vi "Set (SubVI).vi"(8 "Mode":i32, 9 "speed":dbl) -> (0 "Reach?":bool, 1 "Vp":dbl, 2 "Vy":dbl, 3 "Vx":dbl)   [LabVIEW 2017]
uses:
  Projects/Auto control/Inputs.vi
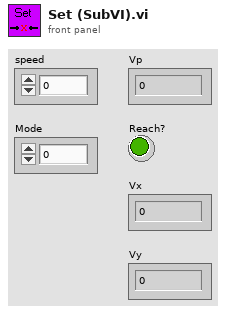
[diagram p1: front panel]
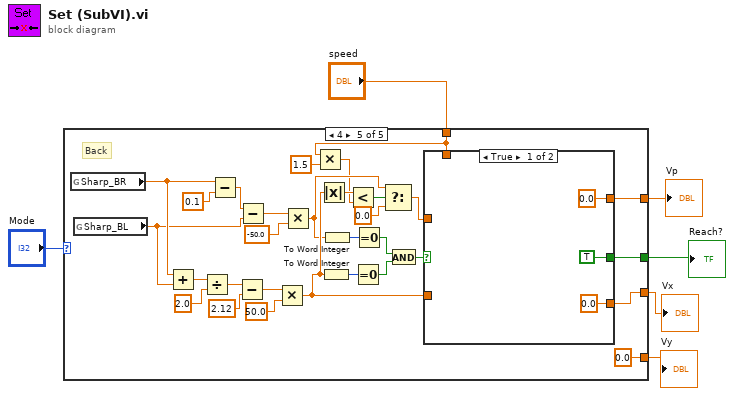
[diagram p0: block diagram]
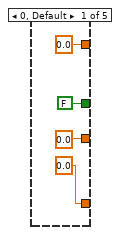
[diagram p2: hidden frame]
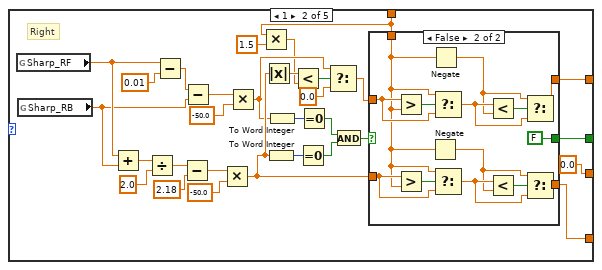
[diagram p3: hidden frame]
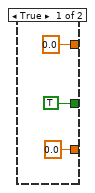
[diagram p4: hidden frame]
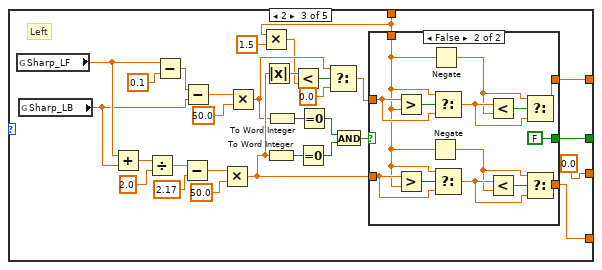
[diagram p5: hidden frame]
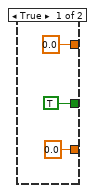
[diagram p6: hidden frame]
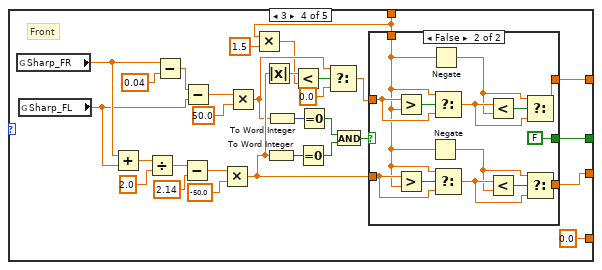
[diagram p7: hidden frame]
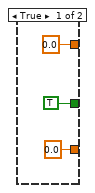
[diagram p8: hidden frame]
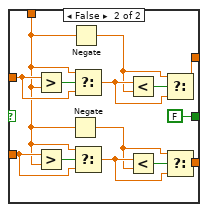
[diagram p9: hidden frame]
diagram:
  n1 = case shown="4" "Mode" {
    tunnel: [0.0 ("speed") w36 w83 w130 w177] -> w2
    tunnel: [0.0 ("speed") 0.0 ("speed") 0.0 ("speed") w106 w153] -> w5
    tunnel: "speed" -> [_ w13 w60 w107 w154]
    tunnel: [FALSE w22 w69 w116 w163] -> w1
    tunnel: [0.0 ("speed") w11 w58 0.0 ("speed") 0.0 ("speed")] -> w6
    frame 0, Default {
    }
    frame 1 {
      # "Right"
      n2 = global read "Inputs.vi" "Sharp_RF"() -> (w35:dbl)
      n3 = global read "Inputs.vi" "Sharp_RB"() -> (w34:dbl)
      n4 = Add(x=w35, y=w34) -> (x+y=w33:dbl)
      n5 = Divide(x=w33, y=2.0) -> (x/y=w31:dbl)
      n6 = Subtract(x=w35, y=0.01) -> (x-y=w40:dbl)
      n7 = Subtract(x=w31, y=2.18) -> (x-y=w29:dbl)
      n8 = Subtract(x=w40, y=w34) -> (x-y=w38:dbl)
      n9 = Multiply(x=w29, y=-50.0) -> (x*y=w18:dbl)
      n10 = Multiply(x=w38, y=-50.0) -> (x*y=w17:dbl)
      n11 = Multiply(x=w13, y=1.5) -> (x*y=w14:dbl)
      n12 = Absolute Value(x=w18) -> (abs(x)=w19:dbl)
      n13 = To Word Integer(number=w18) -> (16bit integer=w26:i16)
      n14 = To Word Integer(number=w17) -> (16bit integer=w27:i16)
      n15 = Less?(x=w19, y=w14) -> (x < y?=w20:bool)
      n16 = Equal To 0?(x=w26) -> (x = 0?=w24:bool)
      n17 = Equal To 0?(x=w27) -> (x = 0?=w23:bool)
      n18 = Select(t=w17, s=w20, f=0.0) -> (s? t:f=w21:dbl)
      n19 = And(x=w23, y=w24) -> (x .and. y?=w25:bool)
      n20 = case shown="False" w25 {
        tunnel: w21 -> [_ w56]
        tunnel: [0.0 ("speed") w52] -> w36
        tunnel: w18 -> [_ w50]
        tunnel: [0.0 ("speed") w46] -> w11
        tunnel: w13 -> [_ w45]
        tunnel: [TRUE FALSE] -> w22
        frame True {
        }
        frame False {
          n21 = Greater?(x=w56, y=w45) -> (0:w57:bool)
          n22 = Greater?(x=w50, y=w45) -> (0:w51:bool)
          n23 = Negate(x=w45) -> (-x=w47:dbl)
          n24 = Negate(x=w45) -> (-x=w53:dbl)
          n25 = Select(t=w45, s=w57, f=w56) -> (s? t:f=w54:dbl)
          n26 = Select(t=w45, s=w51, f=w50) -> (s? t:f=w48:dbl)
          n27 = Less?(x=w54, y=w53) -> (x < y?=w55:bool)
          n28 = Less?(x=w48, y=w47) -> (x < y?=w49:bool)
          n29 = Select(t=w53, s=w55, f=w54) -> (s? t:f=w52:dbl)
          n30 = Select(t=w47, s=w49, f=w48) -> (s? t:f=w46:dbl)
        }
      }
    }
    frame 2 {
      # "Left"
      n31 = global read "Inputs.vi" "Sharp_LF"() -> (w82:dbl)
      n32 = global read "Inputs.vi" "Sharp_LB"() -> (w81:dbl)
      n33 = Add(x=w82, y=w81) -> (x+y=w80:dbl)
      n34 = Divide(x=w80, y=2.0) -> (x/y=w78:dbl)
      n35 = Subtract(x=w82, y=0.1) -> (x-y=w87:dbl)
      n36 = Subtract(x=w78, y=2.17) -> (x-y=w76:dbl)
      n37 = Subtract(x=w87, y=w81) -> (x-y=w85:dbl)
      n38 = Multiply(x=w76, y=50.0) -> (x*y=w65:dbl)
      n39 = Multiply(x=w85, y=50.0) -> (x*y=w64:dbl)
      n40 = Multiply(x=w60, y=1.5) -> (x*y=w61:dbl)
      n41 = Absolute Value(x=w65) -> (abs(x)=w66:dbl)
      n42 = To Word Integer(number=w65) -> (16bit integer=w73:i16)
      n43 = To Word Integer(number=w64) -> (16bit integer=w74:i16)
      n44 = Less?(x=w66, y=w61) -> (x < y?=w67:bool)
      n45 = Equal To 0?(x=w73) -> (x = 0?=w71:bool)
      n46 = Equal To 0?(x=w74) -> (x = 0?=w70:bool)
      n47 = Select(t=w64, s=w67, f=0.0) -> (s? t:f=w68:dbl)
      n48 = And(x=w70, y=w71) -> (x .and. y?=w72:bool)
      n49 = case shown="False" w72 {
        tunnel: w68 -> [_ w103]
        tunnel: [0.0 ("speed") w99] -> w83
        tunnel: w65 -> [_ w97]
        tunnel: [0.0 ("speed") w93] -> w58
        tunnel: w60 -> [_ w92]
        tunnel: [TRUE FALSE] -> w69
        frame True {
        }
        frame False {
          n50 = Greater?(x=w103, y=w92) -> (0:w104:bool)
          n51 = Greater?(x=w97, y=w92) -> (0:w98:bool)
          n52 = Negate(x=w92) -> (-x=w94:dbl)
          n53 = Negate(x=w92) -> (-x=w100:dbl)
          n54 = Select(t=w92, s=w104, f=w103) -> (s? t:f=w101:dbl)
          n55 = Select(t=w92, s=w98, f=w97) -> (s? t:f=w95:dbl)
          n56 = Less?(x=w101, y=w100) -> (x < y?=w102:bool)
          n57 = Less?(x=w95, y=w94) -> (x < y?=w96:bool)
          n58 = Select(t=w100, s=w102, f=w101) -> (s? t:f=w99:dbl)
          n59 = Select(t=w94, s=w96, f=w95) -> (s? t:f=w93:dbl)
        }
      }
    }
    frame 3 {
      # "Front"
      n60 = global read "Inputs.vi" "Sharp_FR"() -> (w129:dbl)
      n61 = global read "Inputs.vi" "Sharp_FL"() -> (w128:dbl)
      n62 = Add(x=w129, y=w128) -> (x+y=w127:dbl)
      n63 = Divide(x=w127, y=2.0) -> (x/y=w125:dbl)
      n64 = Subtract(x=w129, y=0.04) -> (x-y=w134:dbl)
      n65 = Subtract(x=w125, y=2.14) -> (x-y=w123:dbl)
      n66 = Subtract(x=w134, y=w128) -> (x-y=w132:dbl)
      n67 = Multiply(x=w123, y=-50.0) -> (x*y=w112:dbl)
      n68 = Multiply(x=w132, y=50.0) -> (x*y=w111:dbl)
      n69 = Multiply(x=w107, y=1.5) -> (x*y=w108:dbl)
      n70 = Absolute Value(x=w112) -> (abs(x)=w113:dbl)
      n71 = To Word Integer(number=w112) -> (16bit integer=w120:i16)
      n72 = To Word Integer(number=w111) -> (16bit integer=w121:i16)
      n73 = Less?(x=w113, y=w108) -> (x < y?=w114:bool)
      n74 = Equal To 0?(x=w120) -> (x = 0?=w118:bool)
      n75 = Equal To 0?(x=w121) -> (x = 0?=w117:bool)
      n76 = Select(t=w111, s=w114, f=0.0) -> (s? t:f=w115:dbl)
      n77 = And(x=w117, y=w118) -> (x .and. y?=w119:bool)
      n78 = case shown="False" w119 {
        tunnel: w115 -> [_ w150]
        tunnel: [0.0 ("speed") w146] -> w130
        tunnel: w112 -> [_ w144]
        tunnel: [0.0 ("speed") w140] -> w106
        tunnel: w107 -> [_ w139]
        tunnel: [TRUE FALSE] -> w116
        frame True {
        }
        frame False {
          n79 = Greater?(x=w150, y=w139) -> (0:w151:bool)
          n80 = Greater?(x=w144, y=w139) -> (0:w145:bool)
          n81 = Negate(x=w139) -> (-x=w141:dbl)
          n82 = Negate(x=w139) -> (-x=w147:dbl)
          n83 = Select(t=w139, s=w151, f=w150) -> (s? t:f=w148:dbl)
          n84 = Select(t=w139, s=w145, f=w144) -> (s? t:f=w142:dbl)
          n85 = Less?(x=w148, y=w147) -> (x < y?=w149:bool)
          n86 = Less?(x=w142, y=w141) -> (x < y?=w143:bool)
          n87 = Select(t=w147, s=w149, f=w148) -> (s? t:f=w146:dbl)
          n88 = Select(t=w141, s=w143, f=w142) -> (s? t:f=w140:dbl)
        }
      }
    }
    frame 4 {
      # "Back"
      n89 = global read "Inputs.vi" "Sharp_BR"() -> (w176:dbl)
      n90 = global read "Inputs.vi" "Sharp_BL"() -> (w175:dbl)
      n91 = Add(x=w176, y=w175) -> (x+y=w174:dbl)
      n92 = Divide(x=w174, y=2.0) -> (x/y=w172:dbl)
      n93 = Subtract(x=w176, y=0.1) -> (x-y=w181:dbl)
      n94 = Subtract(x=w172, y=2.12) -> (x-y=w170:dbl)
      n95 = Subtract(x=w181, y=w175) -> (x-y=w179:dbl)
      n96 = Multiply(x=w170, y=50.0) -> (x*y=w159:dbl)
      n97 = Multiply(x=w179, y=-50.0) -> (x*y=w158:dbl)
      n98 = Multiply(x=w154, y=1.5) -> (x*y=w155:dbl)
      n99 = Absolute Value(x=w159) -> (abs(x)=w160:dbl)
      n100 = To Word Integer(number=w159) -> (16bit integer=w167:i16)
      n101 = To Word Integer(number=w158) -> (16bit integer=w168:i16)
      n102 = Less?(x=w160, y=w155) -> (x < y?=w161:bool)
      n103 = Equal To 0?(x=w167) -> (x = 0?=w165:bool)
      n104 = Equal To 0?(x=w168) -> (x = 0?=w164:bool)
      n105 = Select(t=w158, s=w161, f=0.0) -> (s? t:f=w162:dbl)
      n106 = And(x=w164, y=w165) -> (x .and. y?=w166:bool)
      n107 = case shown="True" w166 {
        tunnel: w162 -> [_ w197]
        tunnel: [0.0 ("speed") w193] -> w177
        tunnel: w159 -> [_ w191]
        tunnel: [0.0 ("speed") w187] -> w153
        tunnel: w154 -> [_ w186]
        tunnel: [TRUE FALSE] -> w163
        frame True {
        }
        frame False {
          n108 = Greater?(x=w197, y=w186) -> (0:w198:bool)
          n109 = Greater?(x=w191, y=w186) -> (0:w192:bool)
          n110 = Negate(x=w186) -> (-x=w188:dbl)
          n111 = Negate(x=w186) -> (-x=w194:dbl)
          n112 = Select(t=w186, s=w198, f=w197) -> (s? t:f=w195:dbl)
          n113 = Select(t=w186, s=w192, f=w191) -> (s? t:f=w189:dbl)
          n114 = Less?(x=w195, y=w194) -> (x < y?=w196:bool)
          n115 = Less?(x=w189, y=w188) -> (x < y?=w190:bool)
          n116 = Select(t=w194, s=w196, f=w195) -> (s? t:f=w193:dbl)
          n117 = Select(t=w188, s=w190, f=w189) -> (s? t:f=w187:dbl)
        }
      }
    }
  }
  "Reach?" <- w1
  "Vp" <- w2
  "Vx" <- w5
  "Vy" <- w6
